vi "Drain.vi"(8 "Drain":bool, 11 "Fuel Arm":bool) -> (0 "Solenoids":bool[](array[boolean]))   [LabVIEW 2016]
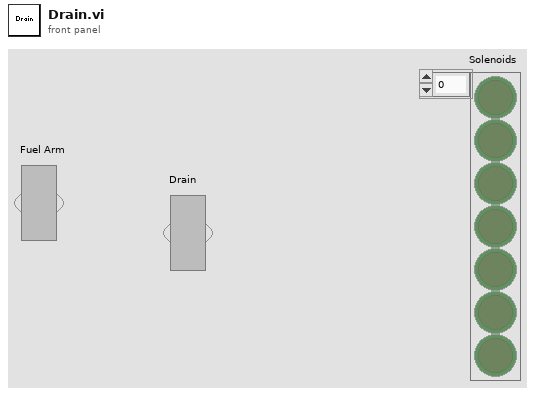
[diagram p1: front panel]
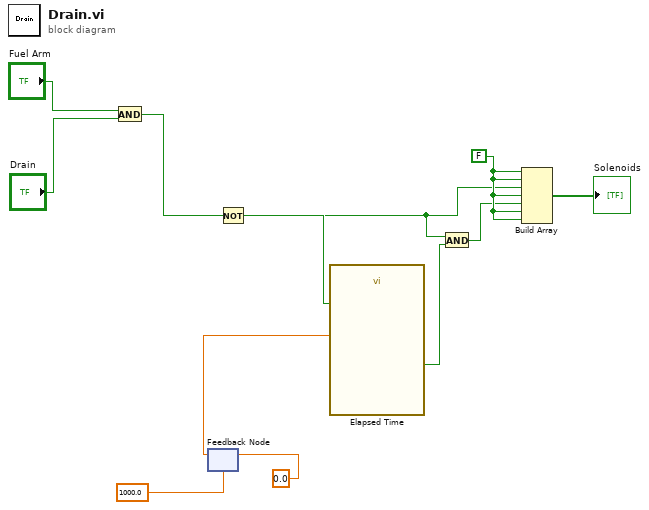
[diagram p0: block diagram]
diagram:
  w4 = FALSE
  n1 = And(x="Fuel Arm", y="Drain") -> (x .and. y?=w1:bool)
  n2 = feedback #1(1000.0) -> (w7:dbl)
  n3 = feedback-in #1(0.0) -> ()
  n4 = Not(x=w1) -> (.not. x?=w6:bool)
  n5 = call "Elapsed Time"("Auto Reset"=w6, "Set Start Time (s)"=w7) -> ("Time has Elapsed"=w2:bool)  [unwired: 10 in, 7 out]
  n6 = And(x=w1, y=w2) -> (x .and. y?=w3:bool)
  n7 = Build Array(w4, w4, w1, w4, w3, w4, w4) -> (→"Solenoids":bool[])
